vi "instr.RelayBD_V03.vi"(6 "测试日志信息":refnum<queue>, 7 "HardWare":enum16{"RelayBD-A", "RelayBD-B", "MCUBD"}(ring), 8 "error in (no error)":errorcluster caption="错误输入（无错误）", 9 "ON/OFF":bool, 10 "Relays":T1(ring), 11 "VISA resource name":refnum<visa-resource-name>="COM1" caption="VISA资源名称") -> (0 "error out":errorcluster caption="错误输出", 3 "OK?":bool)   [LabVIEW 2012, in "Lib_UEL.ATE.lvlib" / "Lib_Instrument.lvlib"]
uses:
  Lib_Instrument.lvlib
  <vilib>/Instr/_visa.llb/VISA Configure Serial Port (Instr).vi
  App/Lib_App.lvlib
panel:
  out "发送字符串":string
  out "返回字符串":string
  out "Return":u8[](array[numeric]) format="%02x"
  in  "timeout (10sec)":u32=1000 caption="超时（10秒）"
  in  "baud rate (9600)":u32=9600 caption="波特率(9600)"
  # "2012-12-18: 确认RelayBD V03可正确工作\n 2013-01-11: 使用队列, 增加测试日志功能.\n 2013-01-16: 增加Set_RelayMode命令,设置是否保存继电器状态"
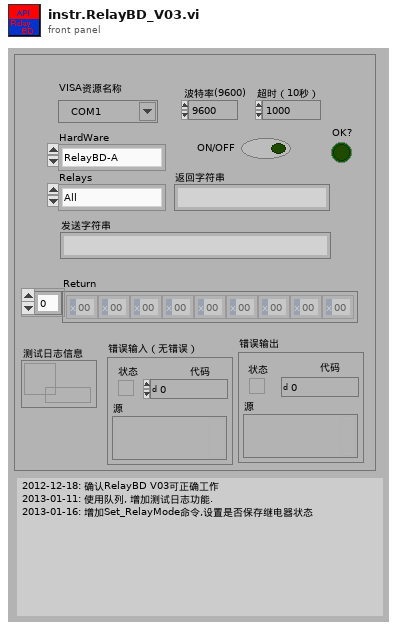
[diagram p1: front panel]
types:
  T1 = enum16{"All", "Group.A", "Group.B", "Relay.A1(BIG)", "Relay.A2", "Relay.A3", "Relay.A4", "Relay.A5", "Relay.A6", "Relay.A7", "Relay.A8(BIG)", "Relay.B1", "Relay.B2", "Relay.B3", "Relay.B4", "Relay.B5", "Relay.B6", "Relay.B7", "Relay.B8", "Check Ver", "Set_RelayMode"}
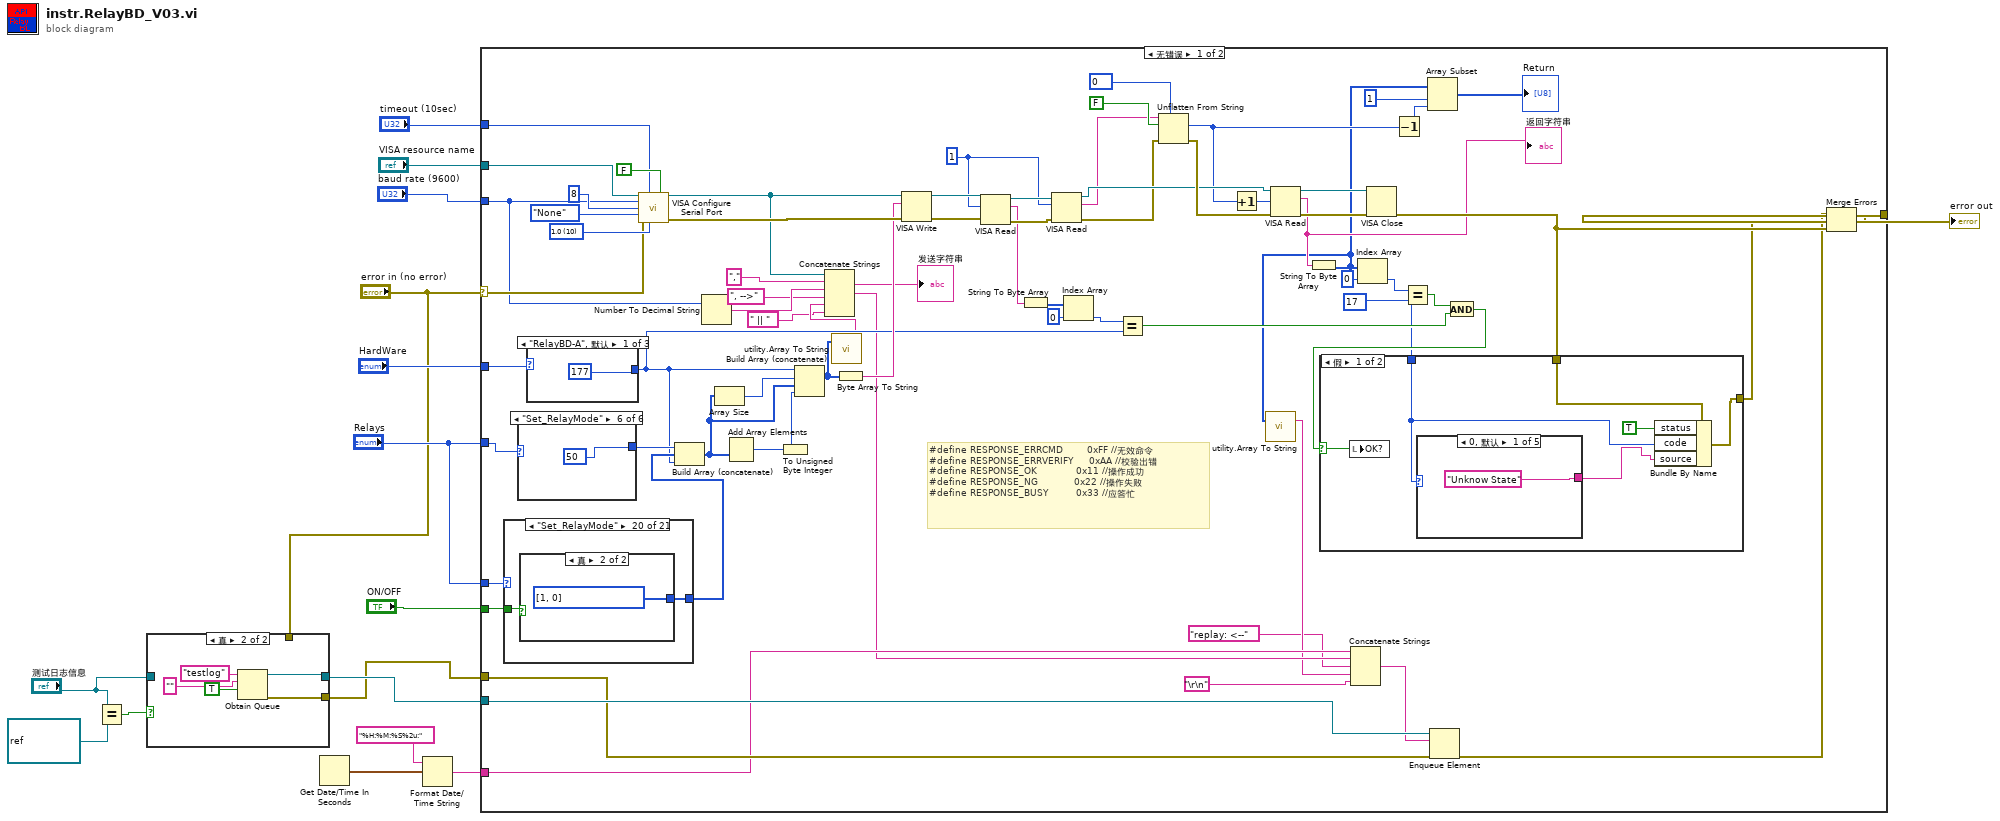
[diagram p0: block diagram]
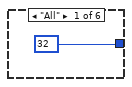
[diagram p3: hidden frame]
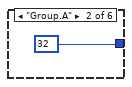
[diagram p4: hidden frame]
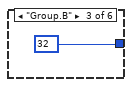
[diagram p5: hidden frame]
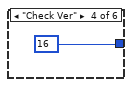
[diagram p6: hidden frame]
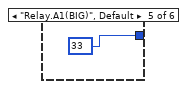
[diagram p7: hidden frame]
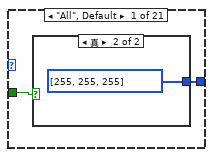
[diagram p8: hidden frame]
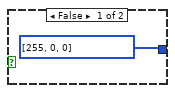
[diagram p9: hidden frame]
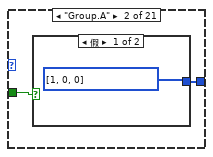
[diagram p10: hidden frame]
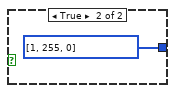
[diagram p11: hidden frame]
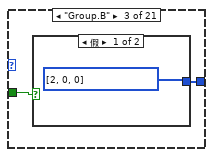
[diagram p12: hidden frame]
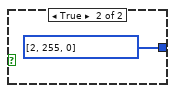
[diagram p13: hidden frame]
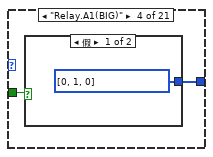
[diagram p14: hidden frame]
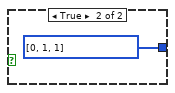
[diagram p15: hidden frame]
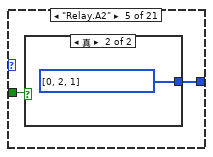
[diagram p16: hidden frame]
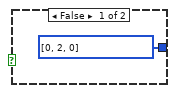
[diagram p17: hidden frame]
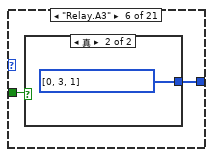
[diagram p18: hidden frame]
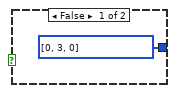
[diagram p19: hidden frame]
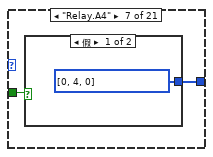
[diagram p20: hidden frame]
diagram:
  n1 = Equal?(x="测试日志信息", y=refnum<queue> refnum) -> (x = y?=w5:bool)
  n2 = case shown="真" w5 {
    tunnel: "测试日志信息" -> [w18 _]
    tunnel: [w18 w23] -> w3
    tunnel: [w17 w22] -> w1
    tunnel: "error in (no error)" -> [w17 _]
    frame False {
    }
    frame True {
      n3 = Obtain Queue(name (unnamed)="testlog" ("名称（未命名）"), element data type="" ("名称（未命名）"), create if not found? (T)=TRUE ("如未找到是否创建？(T)")) -> (queue out=w23:refnum<queue>, error out=w22:errorcluster)  [unwired: 2 in, 1 out]
    }
  }
  n4 = Get Date/Time In Seconds() -> (seconds since 1Jan1904=w8:timestamp)
  n5 = Format Date/Time String(time format string (%c)="%H:%M:%S%2u:" ("时间格式化字符串(%c)"), seconds (now)=w8) -> (date/time string=w7:string)  [unwired: 1 in]
  n6 = case shown="无错误" "error in (no error)" {
    selector: "error in (no error)" -> [w80 w204]
    tunnel: "VISA resource name" -> [w93 _]
    tunnel: [w45 w203] -> w12
    tunnel: "baud rate (9600)" -> [w40 _]
    tunnel: "timeout (10sec)" -> [w86 _]
    tunnel: "HardWare" -> [w79 _]
    tunnel: "Relays" -> [w52 _]
    tunnel: "Relays" -> [w56 _]
    tunnel: "ON/OFF" -> [w55 _]
    tunnel: w1 -> [w33 _]
    tunnel: w3 -> [w34 w202]
    tunnel: w7 -> [w32 w201]
    frame No Error {
      w84 = u16 10 items=["1.0"=10, "1.5"=15, "2.0"=20] ("stop bits (10: 1 bit)")
      w70 = u32 1 ("字节总数")
      # "#define RESPONSE_ERRCMD     \t\t\t0xFF\t//无效命令 \n#define RESPONSE_ERRVERIFY\t\t\t  0xAA\t//校验出错 \n#define RESPONSE_OK           \t\t0x11\t//操作成功 \n#define RESPONSE_NG         \t\t\t0x22\t//操作失败 \n#define RESPONSE_BUSY     \t\t\t\t0x33\t//应答忙"
      n7 = case shown="\"Set_RelayMode\"" w56 {
        tunnel: w55 -> [w101 w105 w109 w113 w117 w121 w125 w129 w133 w137 w141 w145 w149 w153 w157 w161 w165 w169 w173 w177 _]
        tunnel: [w100 w104 w108 w112 w116 w120 w124 w128 w132 w136 w140 w144 w148 w152 w156 w160 w164 w168 w172 w176 u8[] [] ("数组")] -> w54
        frame "All", Default {
          n8 = case shown="真" w101 {
            tunnel: [u8[] [255, 0, 0] ("数组") u8[] [255, 255, 255] ("数组")] -> w100
            frame False {
            }
            frame True {
            }
          }
        }
        frame "Group.A" {
          n9 = case shown="假" w105 {
            tunnel: [u8[] [1, 0, 0] ("数组") u8[] [1, 255, 0] ("数组")] -> w104
            frame False {
            }
            frame True {
            }
          }
        }
        frame "Group.B" {
          n10 = case shown="假" w109 {
            tunnel: [u8[] [2, 0, 0] ("数组") u8[] [2, 255, 0] ("数组")] -> w108
            frame False {
            }
            frame True {
            }
          }
        }
        frame "Relay.A1(BIG)" {
          n11 = case shown="假" w113 {
            tunnel: [u8[] [0, 1, 0] ("数组") u8[] [0, 1, 1] ("数组")] -> w112
            frame False {
            }
            frame True {
            }
          }
        }
        frame "Relay.A2" {
          n12 = case shown="真" w117 {
            tunnel: [u8[] [0, 2, 0] ("数组") u8[] [0, 2, 1] ("数组")] -> w116
            frame False {
            }
            frame True {
            }
          }
        }
        frame "Relay.A3" {
          n13 = case shown="真" w121 {
            tunnel: [u8[] [0, 3, 0] ("数组") u8[] [0, 3, 1] ("数组")] -> w120
            frame False {
            }
            frame True {
            }
          }
        }
        frame "Relay.A4" {
          n14 = case shown="假" w125 {
            tunnel: [u8[] [0, 4, 0] ("数组") u8[] [0, 4, 1] ("数组")] -> w124
            frame False {
            }
            frame True {
            }
          }
        }
        frame "Relay.A5" {
          n15 = case shown="真" w129 {
            tunnel: [u8[] [0, 5, 0] ("数组") u8[] [0, 5, 1] ("数组")] -> w128
            frame False {
            }
            frame True {
            }
          }
        }
        frame "Relay.A6" {
          n16 = case shown="假" w133 {
            tunnel: [u8[] [0, 6, 0] ("数组") u8[] [0, 6, 1] ("数组")] -> w132
            frame False {
            }
            frame True {
            }
          }
        }
        frame "Relay.A7" {
          n17 = case shown="真" w137 {
            tunnel: [u8[] [0, 7, 0] ("数组") u8[] [0, 7, 1] ("数组")] -> w136
            frame False {
            }
            frame True {
            }
          }
        }
        frame "Relay.A8(BIG)" {
          n18 = case shown="假" w141 {
            tunnel: [u8[] [0, 8, 0] ("数组") u8[] [0, 8, 1] ("数组")] -> w140
            frame False {
            }
            frame True {
            }
          }
        }
        frame "Relay.B1" {
          n19 = case shown="真" w145 {
            tunnel: [u8[] [1, 1, 0] ("数组") u8[] [1, 1, 1] ("数组")] -> w144
            frame False {
            }
            frame True {
            }
          }
        }
        frame "Relay.B2" {
          n20 = case shown="假" w149 {
            tunnel: [u8[] [1, 2, 0] ("数组") u8[] [1, 2, 1] ("数组")] -> w148
            frame False {
            }
            frame True {
            }
          }
        }
        frame "Relay.B3" {
          n21 = case shown="真" w153 {
            tunnel: [u8[] [1, 3, 0] ("数组") u8[] [1, 3, 1] ("数组")] -> w152
            frame False {
            }
            frame True {
            }
          }
        }
        frame "Relay.B4" {
          n22 = case shown="假" w157 {
            tunnel: [u8[] [1, 4, 0] ("数组") u8[] [1, 4, 1] ("数组")] -> w156
            frame False {
            }
            frame True {
            }
          }
        }
        frame "Relay.B5" {
          n23 = case shown="真" w161 {
            tunnel: [u8[] [1, 5, 0] ("数组") u8[] [1, 5, 1] ("数组")] -> w160
            frame False {
            }
            frame True {
            }
          }
        }
        frame "Relay.B6" {
          n24 = case shown="假" w165 {
            tunnel: [u8[] [1, 6, 0] ("数组") u8[] [1, 6, 1] ("数组")] -> w164
            frame False {
            }
            frame True {
            }
          }
        }
        frame "Relay.B7" {
          n25 = case shown="真" w169 {
            tunnel: [u8[] [1, 7, 0] ("数组") u8[] [1, 7, 1] ("数组")] -> w168
            frame False {
            }
            frame True {
            }
          }
        }
        frame "Relay.B8" {
          n26 = case shown="假" w173 {
            tunnel: [u8[] [1, 8, 0] ("数组") u8[] [1, 8, 1] ("数组")] -> w172
            frame False {
            }
            frame True {
            }
          }
        }
        frame "Set_RelayMode" {
          n27 = case shown="真" w177 {
            tunnel: [u8[] [0, 0] ("数组") u8[] [1, 0] ("数组")] -> w176
            frame False {
            }
            frame True {
            }
          }
        }
        frame "Check Ver" {
        }
      }
      n28 = case shown="\"Set_RelayMode\"" w52 {
        tunnel: [u8 32 u8 32 u8 32 u8 16 u8 33 u8 50] -> w51
        frame "All" {
        }
        frame "Group.A" {
        }
        frame "Group.B" {
        }
        frame "Check Ver" {
        }
        frame "Relay.A1(BIG)", Default {
        }
        frame "Set_RelayMode" {
        }
      }
      n29 = case shown="\"RelayBD-A\", 默认" w79 {
        tunnel: [u8 177 u8 178 u8 161] -> w42
        frame "RelayBD-A", Default {
        }
        frame "RelayBD-B" {
        }
        frame "MCUBD" {
        }
      }
      n30 = call-poly "VISA Configure Serial Port"("VISA resource name"=w93, "timeout (10sec)"=w86, "Enable Termination\nChar (T)"=FALSE ("Enable Termination\nChar (T)"), "baud rate (9600)"=w40, "data bits (8)"=u16 8, "parity (0:none)"=enum16{"None", "Odd", "Even", "Mark", "Space"}."None", "error in (no error)"=w80, "stop bits (10: 1 bit)"=w84) -> ("VISA resource name out"=w39:refnum<visa-resource-name>, "error out"=w75:errorcluster)  [unwired: 6 in]
      n31 = Build Array (concatenate)(w51, w54, w42) -> (w77:u8[])
      n32 = Number To Decimal String(number=w40) -> (decimal integer string=w38:string)  [unwired: 1 in]
      n33 = Array Size(array=w77) -> (size(s)=w78:i32)
      n34 = Add Array Elements(numeric array=w77) -> (sum=w44:u8)
      n35 = To Unsigned Byte Integer(number=w44) -> (unsigned 8bit integer=w76:u8)
      n36 = Build Array (concatenate)(w42, w78, w77, w76) -> (w41:i32[])
      n37 = call "utility.Array To String.vi"("无符号字节数组"=w41) -> ("命令输出(字符串)"=w36:string)  [unwired: 1 in, 1 out]
      n38 = Concatenate Strings(w39, "," ("字符串"), w38, ", -->" ("字符串"), w36, " || " ("字符串")) -> (w31:string)
      "发送字符串" <- w31
      n39 = Byte Array To String(unsigned byte array=w41) -> (string=w74:string)
      n40 = VISA Write(VISA resource name=w39, write buffer=w74, error in (no error)=w75) -> (VISA resource name out=w91:refnum<visa-resource-name>, error out=w90:errorcluster)  [unwired: 1 out]
      n41 = VISA Read(VISA resource name=w91, byte count=w70, error in (no error)=w90) -> (VISA resource name out=w71:refnum<visa-resource-name>, read buffer=w66:string, error out=w72:errorcluster)  [unwired: 1 out]
      n42 = String To Byte Array(string=w66) -> (unsigned byte array=w65:u8[])
      n43 = VISA Read(VISA resource name=w71, byte count=w70, error in (no error)=w72) -> (VISA resource name out=w69:refnum<visa-resource-name>, read buffer=w67:string, error out=w68:errorcluster)  [unwired: 1 out]
      n44 = Index Array(array=w65, index=0 ("索引")) -> (element=w63:u8)
      n45 = Equal?(x=w63, y=w42) -> (x = y?=w59:bool)
      n46 = Unflatten From String(type=u8 0, binary string=w67, data includes array or string size? (T)=FALSE ("数据中包含数组或字符串大小？(T)"), error in (no error)=w68) -> (value=w48:u8, error out=w81:errorcluster)  [unwired: 1 in, 1 out]
      n47 = Increment(x=w48) -> (x+1=w73:u8)
      n48 = VISA Read(VISA resource name=w69, byte count=w73, error in (no error)=w81) -> (VISA resource name out=w89:refnum<visa-resource-name>, read buffer=w43:string, error out=w88:errorcluster)  [unwired: 1 out]
      "返回字符串" <- w43
      n49 = String To Byte Array(string=w43) -> (unsigned byte array=w30:u8[])
      n50 = call "utility.Array To String.vi"("无符号字节数组"=w30) -> ("命令输出(字符串)"=w28:string)  [unwired: 1 in, 1 out]
      n51 = Concatenate Strings(w32, w31, "replay: <--" ("字符串"), w28, "\r\n") -> (w26:string)
      n52 = Index Array(array=w30, index=0 ("索引")) -> (element=w49:u8)
      n53 = VISA Close(VISA resource name=w89, error in (no error)=w88) -> (error out=w47:errorcluster)
      n54 = Decrement(x=w48) -> (x-1=w50:u8)
      n55 = Equal?(x=w49, y=u8 17) -> (x = y?=w60:bool)
      n56 = Array Subset(array=w30, index=1 ("索引"), length=w50) -> (→"Return":u8[])
      n57 = Enqueue Element(queue=w34, element=w26, error in (no error)=w33) -> (error out=w25:errorcluster)  [unwired: 1 in, 2 out]
      n58 = And(x=w60, y=w59) -> (x .and. y?=w58:bool)
      n59 = case shown="假" w58 {
        selector: w58 -> [w186 w193]
        tunnel: [w183 w192] -> w46
        tunnel: w47 -> [w185 w192]
        tunnel: w49 -> [w182 _]
        frame False {
          n60 = local write "OK?"(w186) -> ()
          n61 = case shown="0, 默认" w182 {
            tunnel: ["Unknow State" ("source") "Wrong CMD" ("source") "Verify Err" ("source") "Fail" ("source") "Busy" ("source")] -> w181
            frame 0, Default {
            }
            frame 255 {
            }
            frame 170 {
            }
            frame 34 {
            }
            frame 35 {
            }
          }
          n62 = Bundle By Name(cluster=w185, "status"=TRUE, "code"=w182, "source"=w181) -> (w183:errorcluster)
        }
        frame True {
          "OK?" <- w193
        }
      }
      n63 = Merge Errors(w25, w46, w47) -> (w45:errorcluster)
    }
    frame Error {
      n64 = Concatenate Strings(w201, "ERR Input." ("字符串"), "\r\n") -> (w198:string)
      n65 = Enqueue Element(queue=w202, element=w198, error in (no error)=errorcluster {"status"=FALSE, "code"=0, "source"=""} ("错误输入（无错误）")) -> (error out=w205:errorcluster)  [unwired: 1 in, 2 out]
      n66 = Wait (ms)(milliseconds to wait=u32 5 ("等待时间（毫秒）")) -> ()  [unwired: 1 out]
      n67 = Merge Errors(w204, w205) -> (w203:errorcluster)
      n68 = local write "OK?"(FALSE ("OK?")) -> ()
    }
  }
  "error out" <- w12
